vi "Update Nagler.vi"(8 "error in (no error)":errorcluster, 11 "TCP Stream in":refnum<class "TCP Stream.lvclass">) -> (0 "error out":errorcluster, 3 "TCP Stream out":refnum<class "TCP Stream.lvclass">)   [LabVIEW 2020, in "TCP Stream.lvclass"]
uses:
  TCP Stream.lvclass
  TCP Stream.lvclass/TCP Stream.ctl
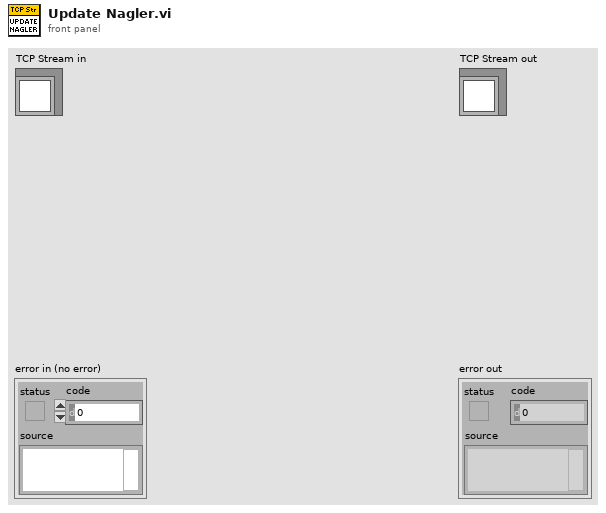
[diagram p1: front panel]
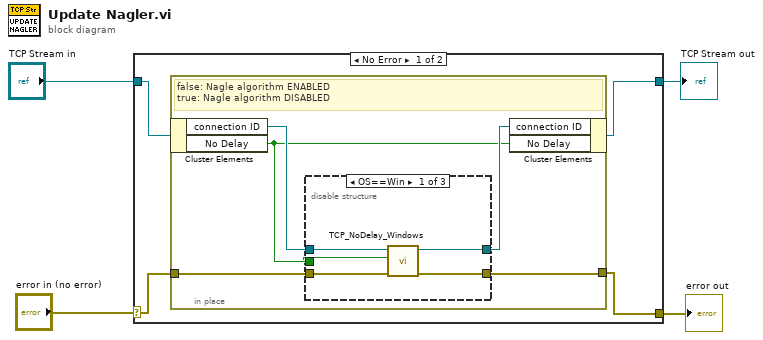
[diagram p0: block diagram]
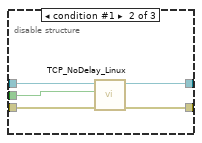
[diagram p2: hidden frame]
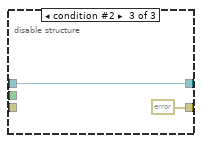
[diagram p3: hidden frame]
diagram:
  n1 = case shown="No Error" "error in (no error)" {
    selector: "error in (no error)" -> [w8 w27]
    tunnel: [w7 w27] -> w3
    tunnel: [w5 w26] -> w1
    tunnel: "TCP Stream in" -> [w6 w26]
    frame No Error {
      n2 = in-place {
        in-place-border: w8 -> [w12]
        in-place-border: [w11] -> w7
        # "false: Nagle algorithm ENABLED\ntrue: Nagle algorithm DISABLED"
        n3 = in-place-cluster #1(w6) -> ("connection ID"=w13:refnum<k5>, "No Delay"=w9:bool)
        n4 = disable-structure shown="OS==Win" {
          disable-tunnel: w13 -> [w18 w23 w25]
          disable-tunnel: w9 -> [w17 w22 _]
          disable-tunnel: w12 -> [w16 w21 _]
          disable-tunnel: [w15 w20 errorcluster {"status"=TRUE, "code"=0, "source"="SO not supported."} ("error out")] -> w11
          disable-tunnel: [w14 w19 w25] -> w10
          frame condition #0 (active) {
            n5 = call "TCP_NoDelay_Windows.vi"("error in (no error)"=w16, "TCP_NODELAY (true)"=w17, "connID"=w18) -> ("error out"=w15:errorcluster, "connID 2"=w14:refnum<k5>)  [unwired: 3 in]
          }
          frame condition #1 {
            n6 = call "TCP_NoDelay_Linux.vi"("error in (no error)"=w21, "TCP_NODELAY (true)"=w22, "connID"=w23) -> ("error out"=w20:errorcluster, "connID 2"=w19:refnum<k5>)  [unwired: 3 in]
          }
          frame condition #2 {
          }
        }
        n7 = in-place-cluster #1("connection ID"=w10, "No Delay"=w9) -> (w5:refnum<class "TCP Stream.lvclass">)
      }
    }
    frame Error {
    }
  }
  "error out" <- w3
  "TCP Stream out" <- w1
